vi "PowerMonitoring.vi"() -> ()   [LabVIEW 2014]
panel:
  out "cluster":T1
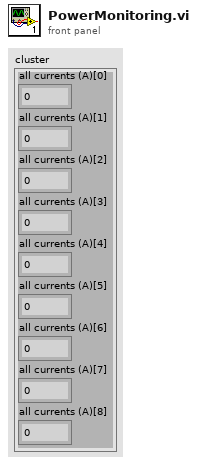
[diagram p1: front panel]
types:
  T1 = cluster{"all currents (A)[0]":dbl, "all currents (A)[1]":dbl, "all currents (A)[2]":dbl, "all currents (A)[3]":dbl, "all currents (A)[4]":dbl, "all currents (A)[5]":dbl, "all currents (A)[6]":dbl, "all currents (A)[7]":dbl, "all currents (A)[8]":dbl}
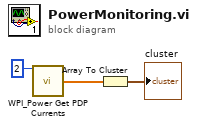
[diagram p0: block diagram]
diagram:
  n1 = call <vilib>:"WPI_Power Get PDP Currents.vi"("Power Distribution Panel (0)"=u8 2) -> ("all currents (A)"=w3:dbl[])  [unwired: 12 in, 2 out]
  n2 = Array To Cluster(array=w3) -> (cluster=→"cluster":T1)
